vi "SID4.vi"() -> ()   [LabVIEW 2013]
uses:
  Program Files (x86)/SID4_SDK/SDKSID4_Types.llb/Refnum SDKSID4 session.ctl
  Shared/GUI_Template/GUI_master/tcp new data cluster.ctl
  <vilib>/vision/Image Controls.llb/IMAQ Image.ctl
  <vilib>/vision/NI_Vision_Development_Module.lvlib
  Shared/GUI_Template/GUI_master/tcp_new_data_event.ctl
  Program Files (x86)/SID4_SDK/SDKSID4_Types.llb/SDKSID4_Analysis info.ctl
  Program Files (x86)/SID4_SDK/SDKSID4_Types.llb/SDKSID4_Camera info.ctl
  Program Files (x86)/SID4_SDK/SDKSID4_Types.llb/SDKSID4_ImageCameraSize.ctl
panel:
  out "ROI Descriptor out":T1={"Global Rectangle"=[10, 10, 200, 200], "Contours"=[{"ID"=enum."External", "Type"=4, "Coordinates"=[10, 10, 200, 200]}]} {"Contours"."Type" items=["No Selection", "Point", "Line", "Rectangle", "Oval", "Polygon", "Free", "Annulus", "Unused2", "Unused3", "Broken Line", "Free Hand Line", "Rotated Rectangle"]}
  in  "pattern":string="*.png"
  in  "analyze folder":bool caption="sdfd"
  out "filenames":string[](array[string])
  in  "Folder to analyze":path=path "C:/Program Files (x86)/SID4_SDK/Examples/Mask files/Mask1.msk"
  in  "file?":bool caption="file (T) Live (F)"
  in  "save raw":bool caption="saves the intensity image retrieved from GEECS"
  in  "save measurement":bool caption="saves the recovered intensity and phase"
  in  "analyze":bool caption="analyzes the phase on either a file or the live image from GEECS"
  in  "continuous analysis":bool
  in  "Tab Control":T2(tab)
  in  "Profile path":path=path "C:/Users/loasis/Documents/000 Labview Local/Developers Version/Interface/GUI_SID4/profiles/SID4-034d default profile/SID4-034d default profile.txt"
  in  "Interferogram path":path=path "H:/data/p2/Y2014/09-Sep/14_0930/scans/Scan003/P2-phasics/Scan003_P2-phasics_047.png"
  in  "Reference Interferogram path":path=path "H:/data/p2/Y2014/09-Sep/14_0930/scans/Scan003/P2-phasics/Scan003_P2-phasics_001.png"
  in  "change reference":bool
  out "Saved Phase file":path
  out "Intensity file":path
  in  "GUIdevice 1":string="P2-phasics"
  in  "Tmp path":path=path "C:/Program Files (x86)/SID4_SDK/Examples/Interferograms/delete.tif"
  out "UnwrappingAlgoritm":u16(ring) items=["Basic", "Goldstein", "Lp-Norm"]
  out "UnwrappingOptions":u8[](array[numeric])
  out "Adv_Activation out":bool
  out "Adv_Niter":u16=10 caption="AdvAnalyse_# iterations out"
  out "Adv_MSE_Threshold":sgl=0.001 caption="AdvAnalyse_threshold out" format="%#.3e"
  in  "UnwrappingAlgoritm IN":u16(ring) items=["Basic", "Goldstein", "Lp-Norm"]
  in  "UnwrappingOptions IN":u8[](array[numeric])=[0, 0, 0, 0]
  in  "Adv_Activation in":bool
  in  "Adv_Niter 2":u16=10 caption="AdvAnalyse_# iterations in"
  in  "Adv_MSE_Threshold 2":sgl=0.001 caption="AdvAnalyse_threshold in" format="%#.3e"
  in  "change advanced parameters":bool caption="sdfd"
  out "image::1":T3(plugin-control) caption="Intensity"
  out "phasics-int1":T3(plugin-control)
  in  "change mask":bool
  in  "Tab Control 2":enum32{"Phase int graph", "Phase vision image"}(tab)
  out "PHASE":sgl[][](graph)
  out "phaseplot":T3(plugin-control)
  in  "Tab Control 3":enum32{"Intensity graph", "Phase lineout"}(tab)
  out "INTENSITY":sgl[][](graph)
  out "Line Profile":cluster{"x0":sgl, "dx":sgl, "Pixels Line":sgl[]}(graph)
  out "Line Information":T4 {"Standard Deviation" format="%#.2f"; "Mean" format="%#.2f"}
  out "SDKVersion":string
  out "Analysis info":T5
  out "Camera info":T6
  out "SNPhasics":string
  out "UserProfileDirectory":string
  out "UserProfile_LastReference":string
  out "UserProfileDescription":string
  out "UserProfile_File":string
  out "UserProfileName":string
  out "ImageCameraSize":T7
  in  "stop":bool
  out "tcp data event":T8
  out "error IO 2":errorcluster
  in  "MASK":T9(tab)
  in  "Mask path":path=path "C:/Program Files (x86)/SID4_SDK/Examples/Mask files/Mask1.msk"
  in  "ROI Descriptor IN":T1={"Global Rectangle"=[10, 10, 200, 200], "Contours"=[{"ID"=enum."External", "Type"=4, "Coordinates"=[10, 10, 200, 200]}]} {"Contours"."Type" items=["No Selection", "Point", "Line", "Rectangle", "Oval", "Polygon", "Free", "Annulus", "Unused2", "Unused3", "Broken Line", "Free Hand Line", "Rotated Rectangle"]}
  out "Current State":string
  # "Ensure paths in the profile path are correct to begin with or this program will not work!!!"
  # "Short term:\nfolder analysis\nrms deviation\n\n\nLong term:\nMode analysis\nAuto ROI based on intensity"
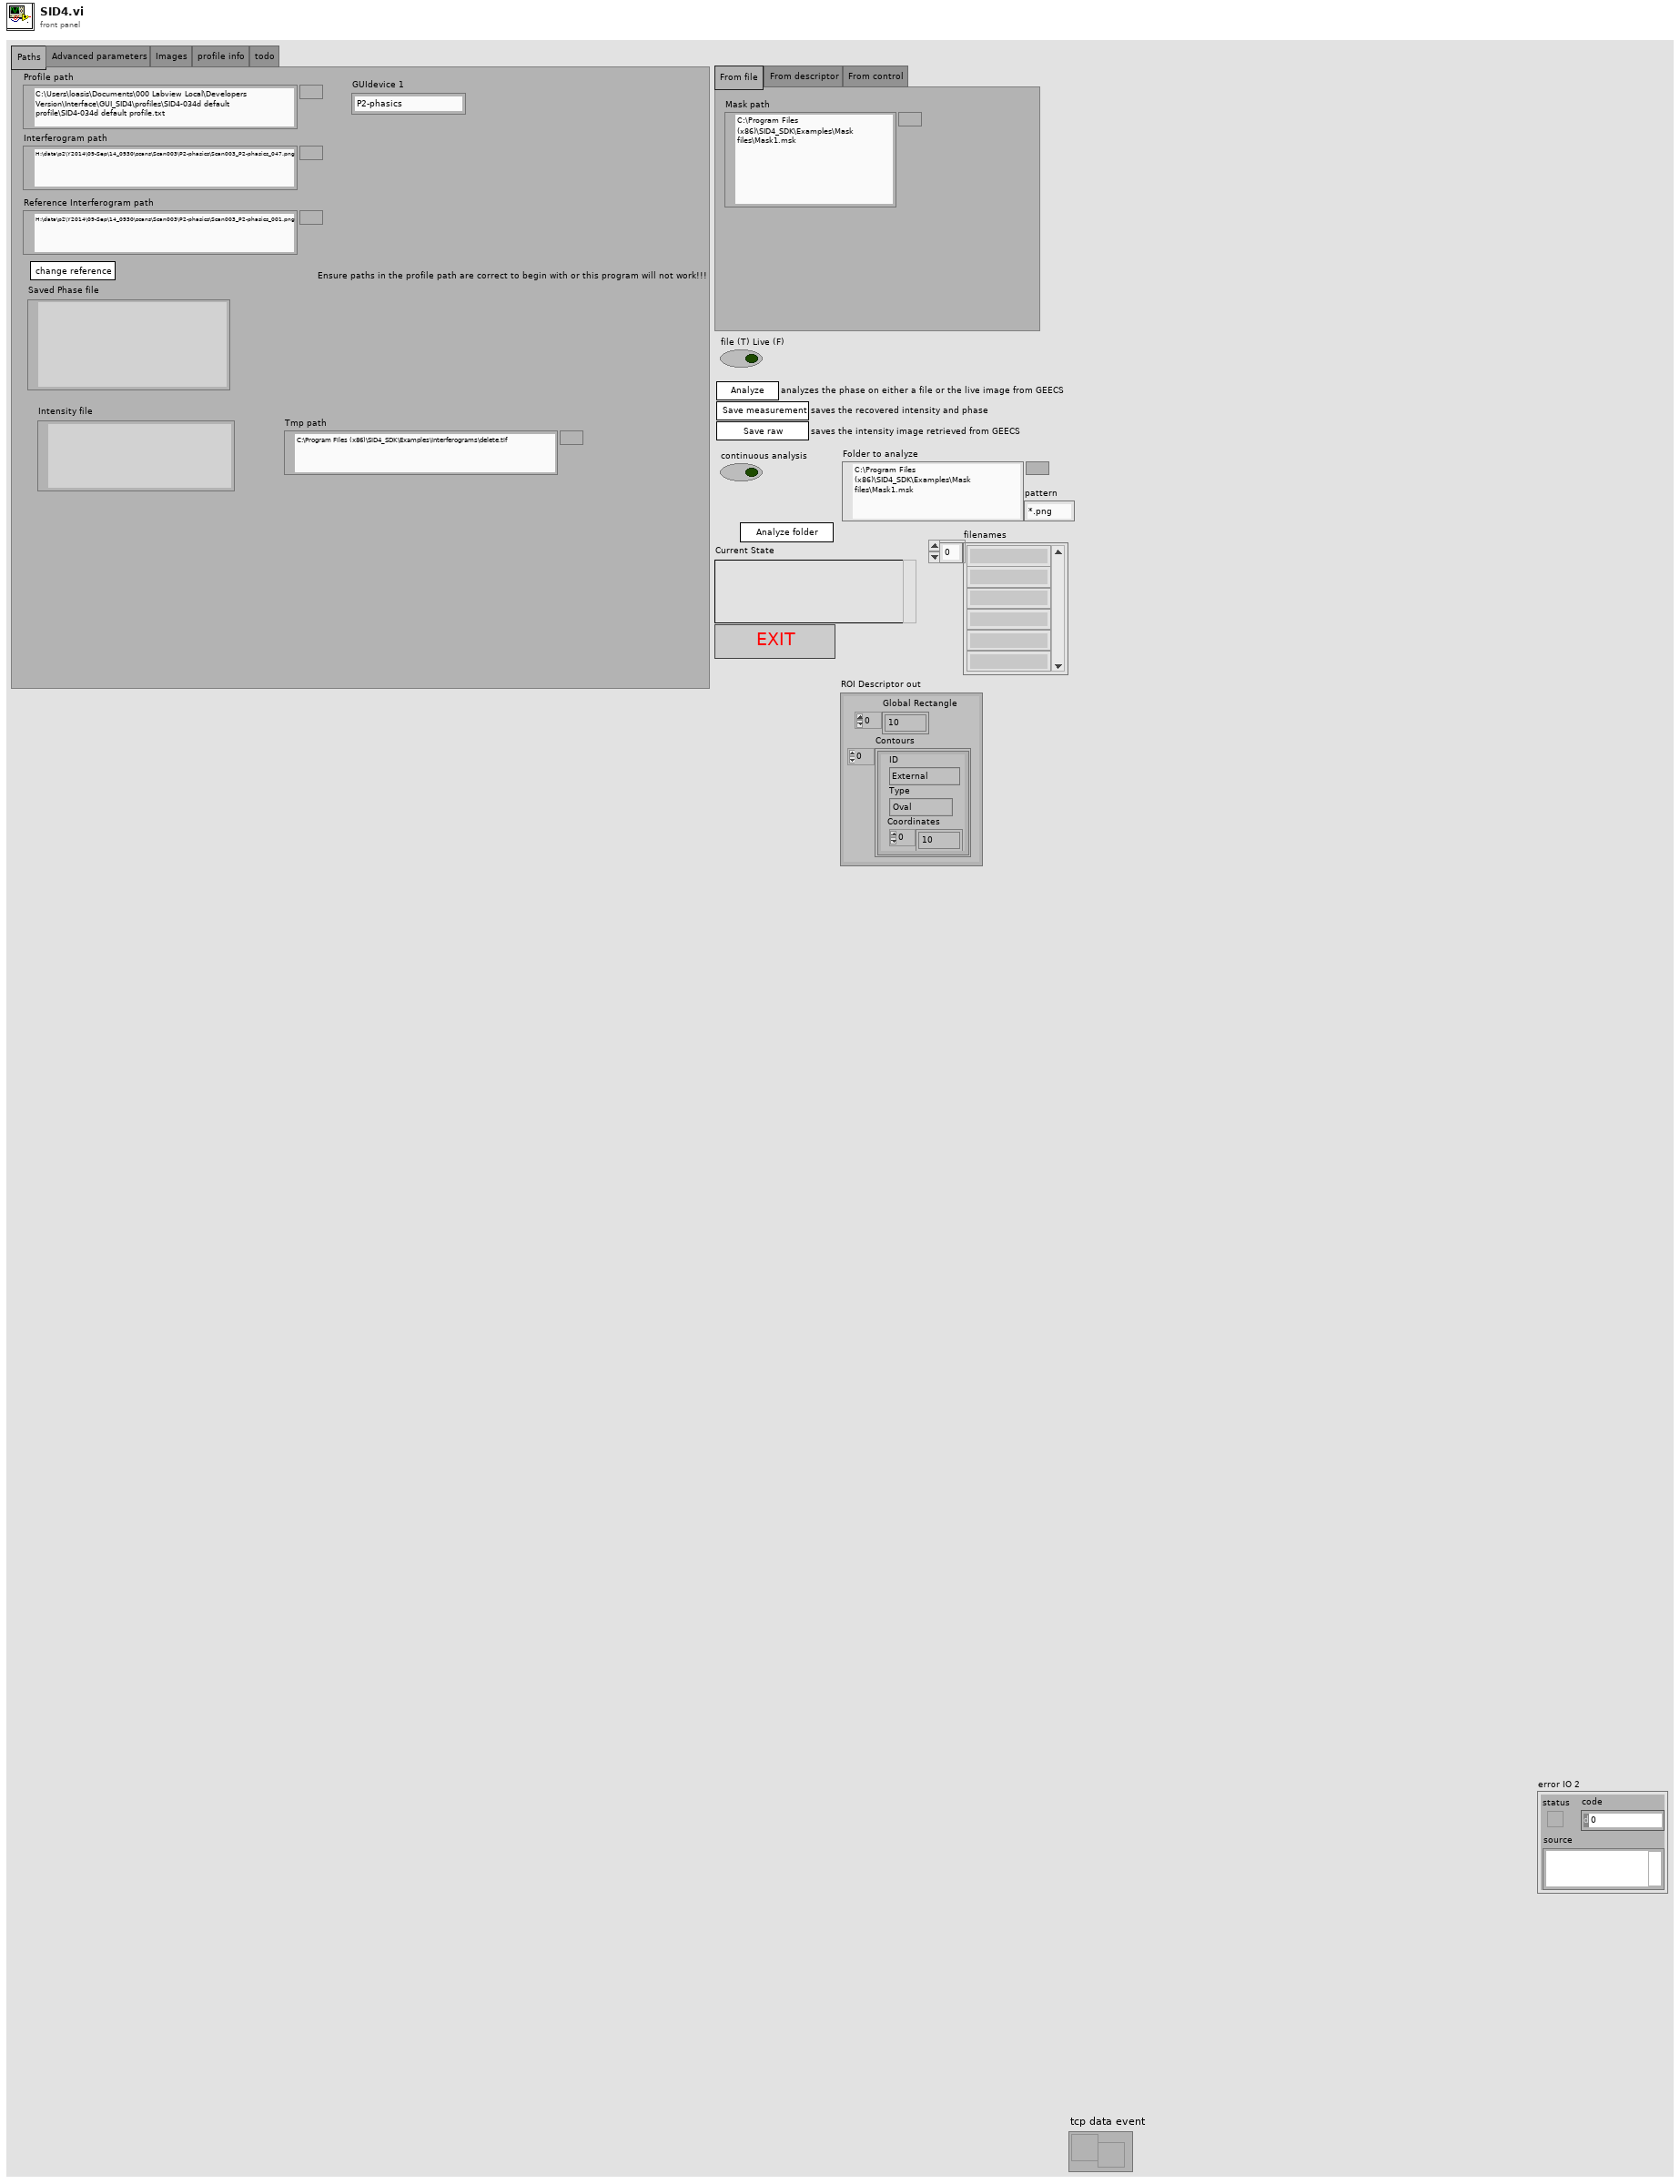
[diagram p1: front panel]
types:
  T1 = cluster{"Global Rectangle":i32[], "Contours":cluster{"ID":enum32{"External", "Internal"}, "Type":u32, "Coordinates":i32[]}[]}
  T2 = enum32{"Paths", "Advanced parameters", "Images", "profile info", "todo"}
  T3 = typedef "IMAQ Image.ctl" = refnum<image>
  T4 = cluster{"Minimum":sgl, "Maximum":sgl, "Mean":sgl, "Standard Deviation":sgl, "Count":i32}
  T5 = typedef "SDKSID4_Analysis info.ctl" = cluster{"Grating position (mm)":dbl, "wavelength (nm)":dbl, "Remove background image":bool, "PhaseSize_width":i32, "PhaseSize_Height":i32}
  T6 = typedef "SDKSID4_Camera info.ctl" = cluster{"Frame rate":i32, "Trigger mode":u32, "Gain":i32, "Exposure time":u32, "PixelSize(µm)":sgl, "NumberOfCameraRecorded":u8}
  T7 = typedef "SDKSID4_ImageCameraSize.ctl" = cluster{"nRow":i32, "nCol":i32}
  T8 = typedef "tcp_new_data_event.ctl" = refnum<user-event>
  T9 = enum32{"From file", "From descriptor", "From control"}
  T10 = typedef "tcp new data cluster.ctl" = cluster{"EventEnum":enum16{"new data", "connection status update"}, "Device name":string}
  T11 = enum32{"invalid app kind", "Development System", "Run Time System", "Student Edition", "Embedded LabVIEW", "Evaluation", "Custom"}
  T12 = typedef "Refnum SDKSID4 session.ctl" = refnum<k1>
  T13 = cluster{"Core":cluster{"Current VI Reference":refnum<vi>, "Close Panel on Exit?":bool}, "SDKSID4 sessionID":T12, "Interferogram path":path, "INTENSITY":sgl[][], "PHASE":sgl[][], "File paths":path[]}
  T14 = enum32{"Invalid", "Standard", "Closed", "Hidden", "Minimized", "Maximized"}
  T15 = typedef "Image Type" = u32
  T16 = cluster{"Global Rectangle":i32[], "Contours":cluster{"Contour Type":u32, "ROI Type":u32, "Points":i32[]}[]}
  T17 = cluster{"Min":sgl, "Max":sgl, "Mean":sgl, "Std Dev":sgl, "Count":i32}
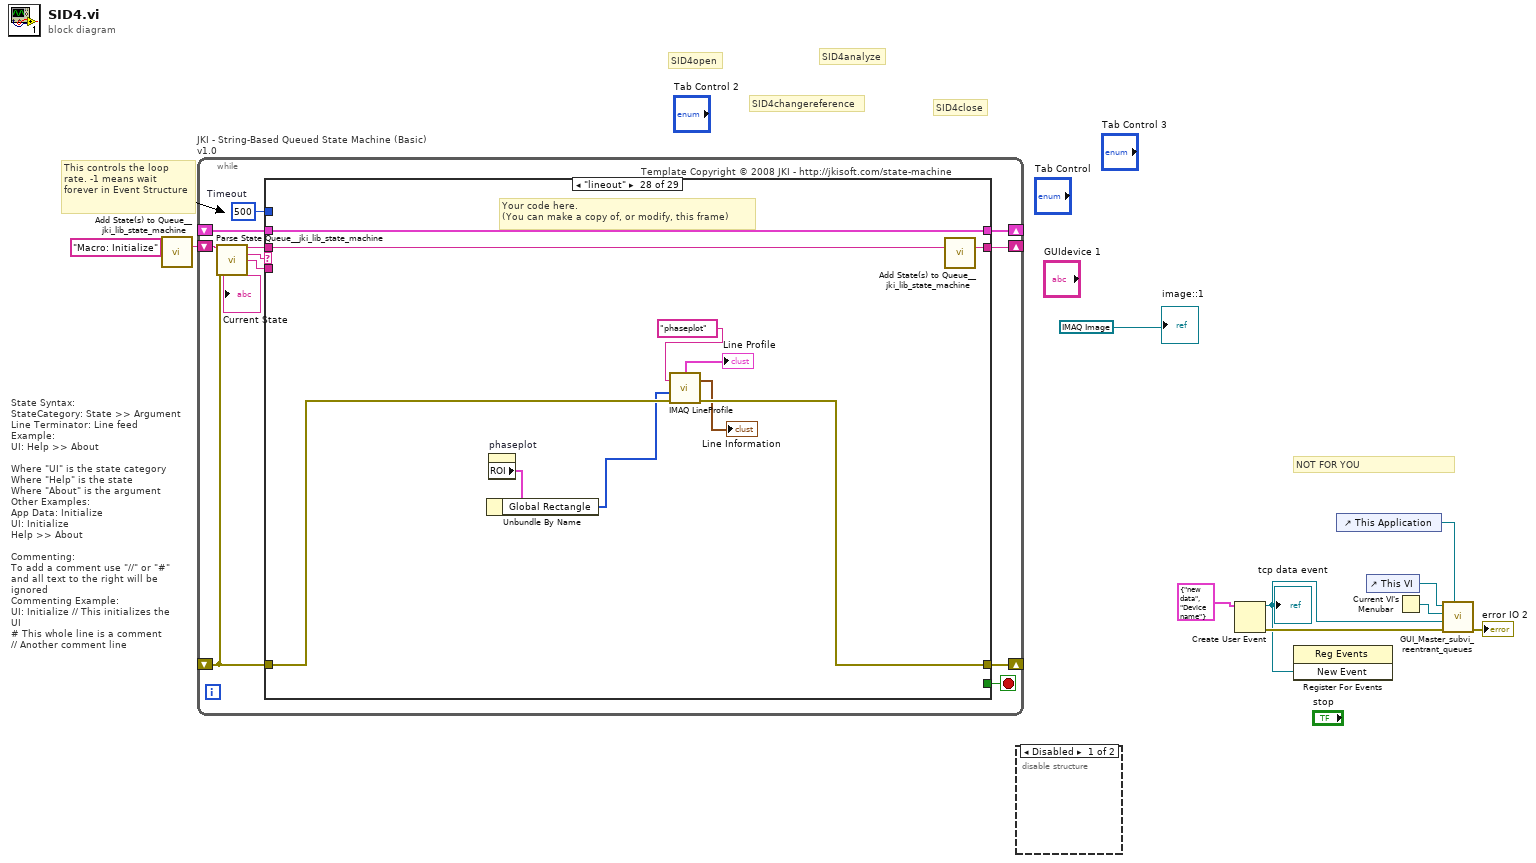
[diagram p0: block diagram]
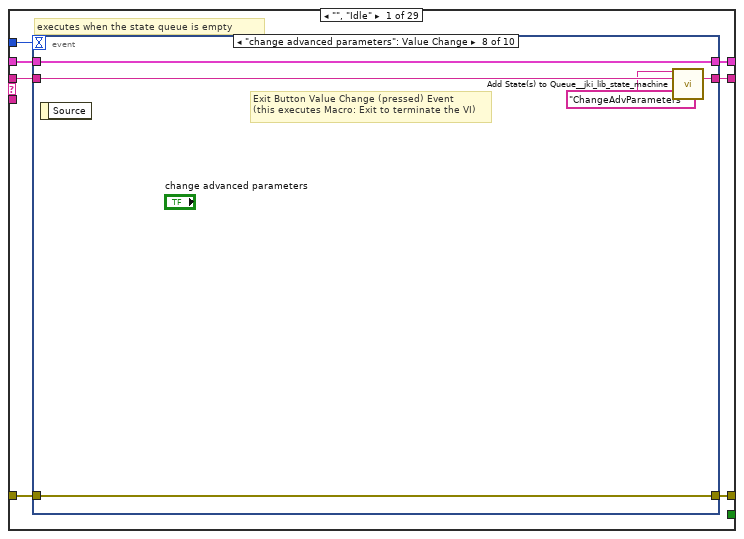
[diagram p3: hidden frame]
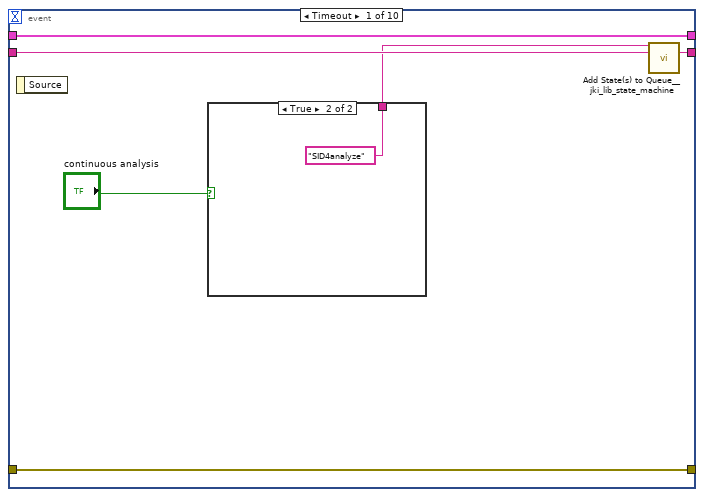
[diagram p4: hidden frame]
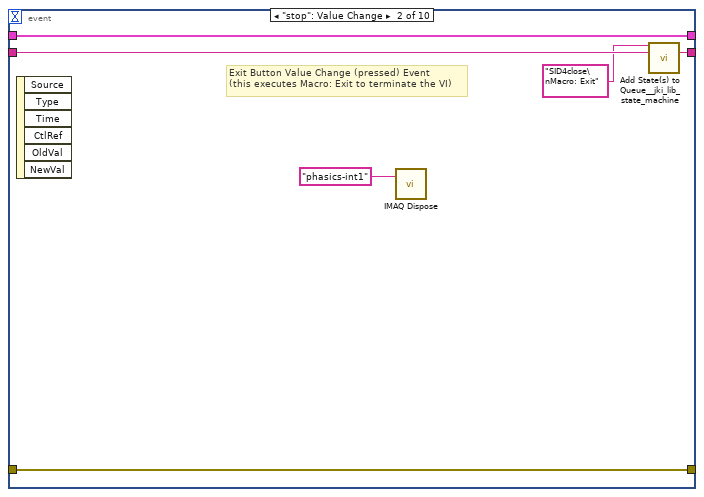
[diagram p6: hidden frame]
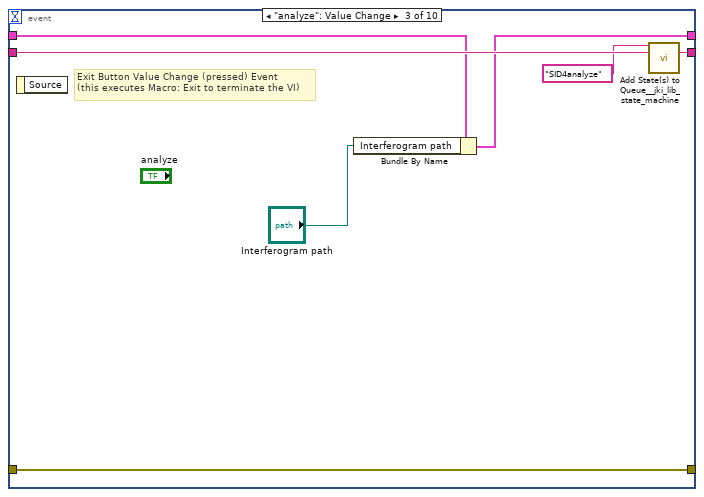
[diagram p7: hidden frame]
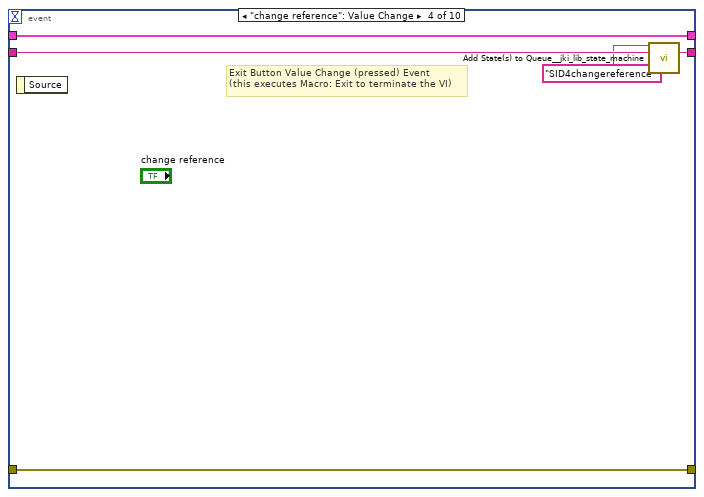
[diagram p8: hidden frame]
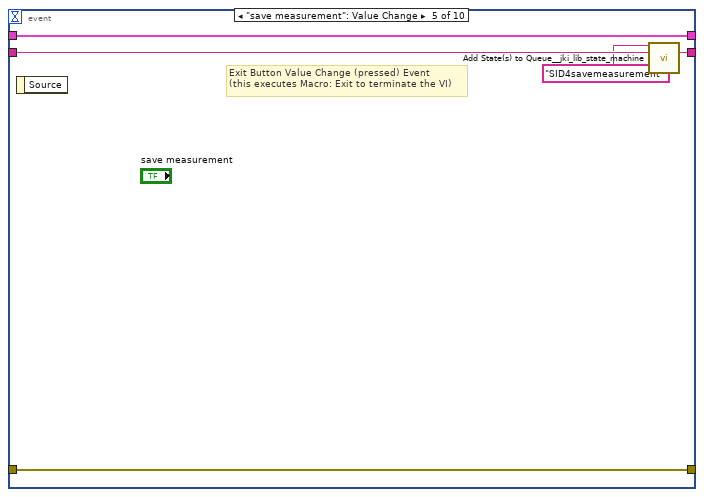
[diagram p9: hidden frame]
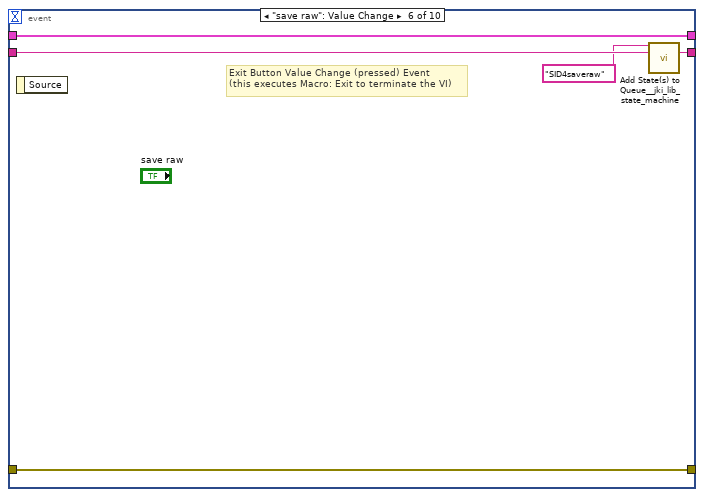
[diagram p10: hidden frame]
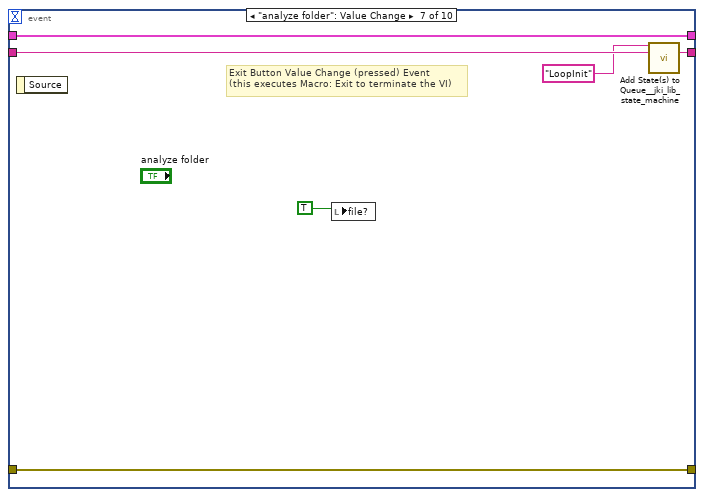
[diagram p11: hidden frame]
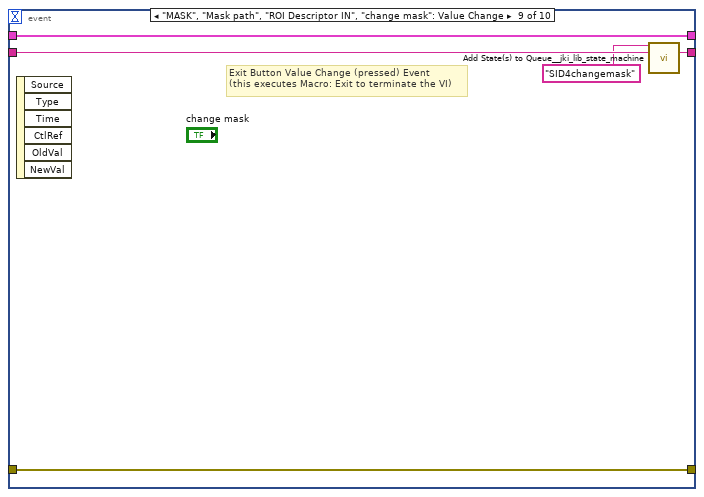
[diagram p12: hidden frame]
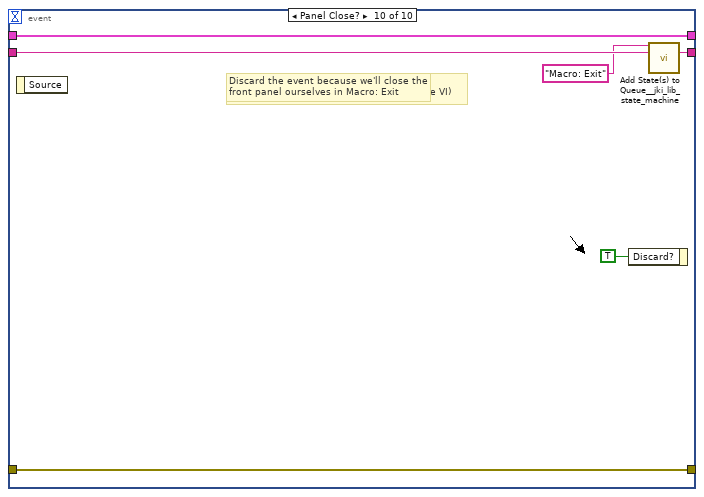
[diagram p13: hidden frame]
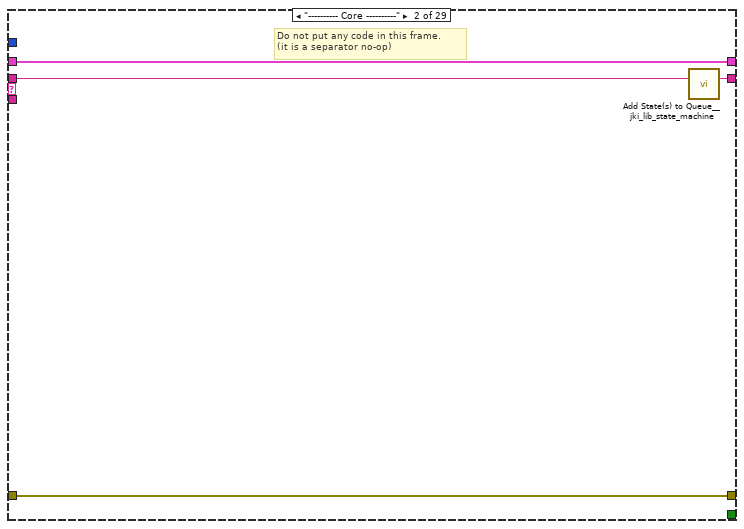
[diagram p14: hidden frame]
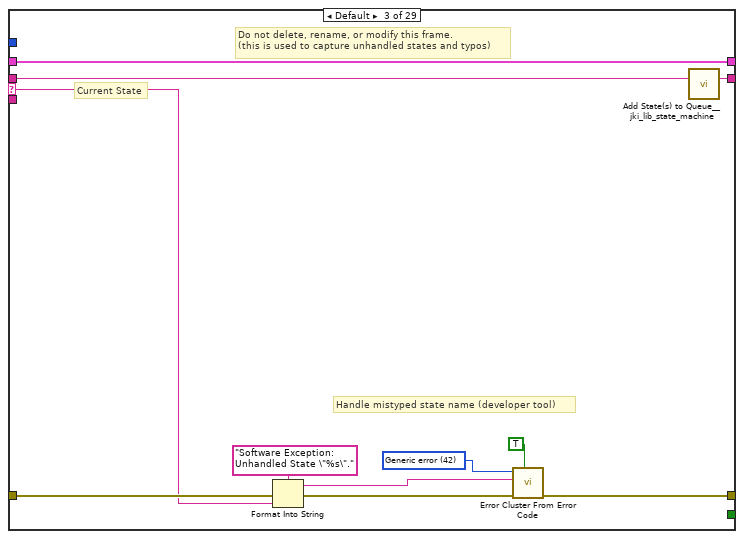
[diagram p15: hidden frame]
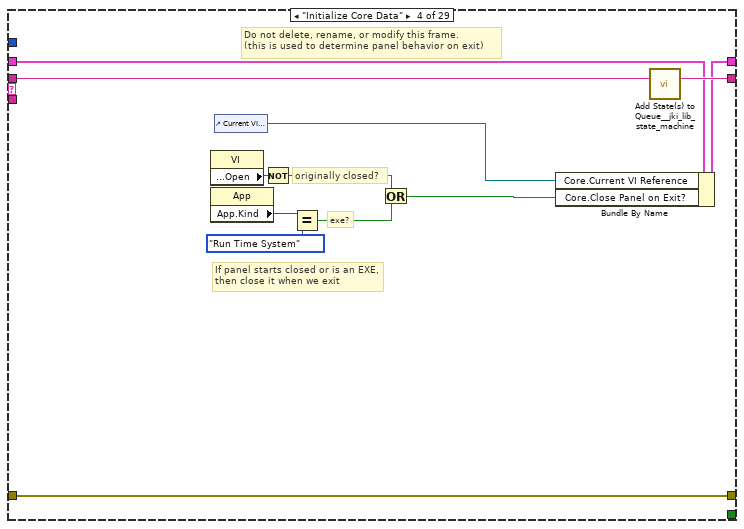
[diagram p16: hidden frame]
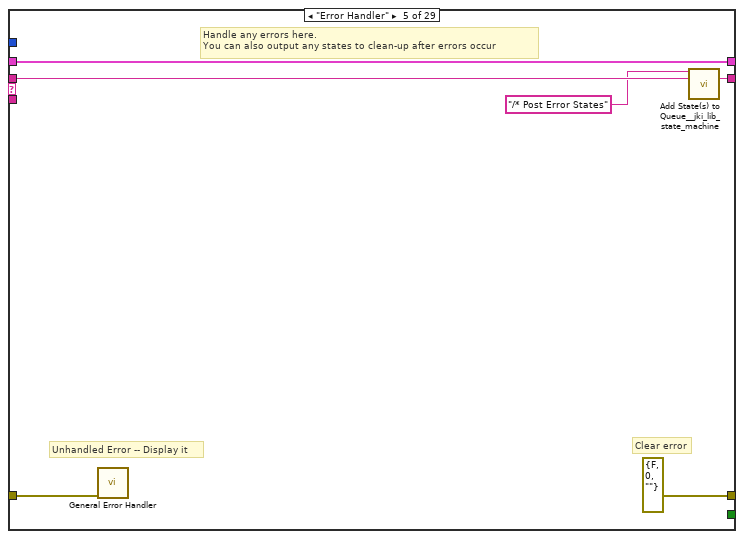
[diagram p17: hidden frame]
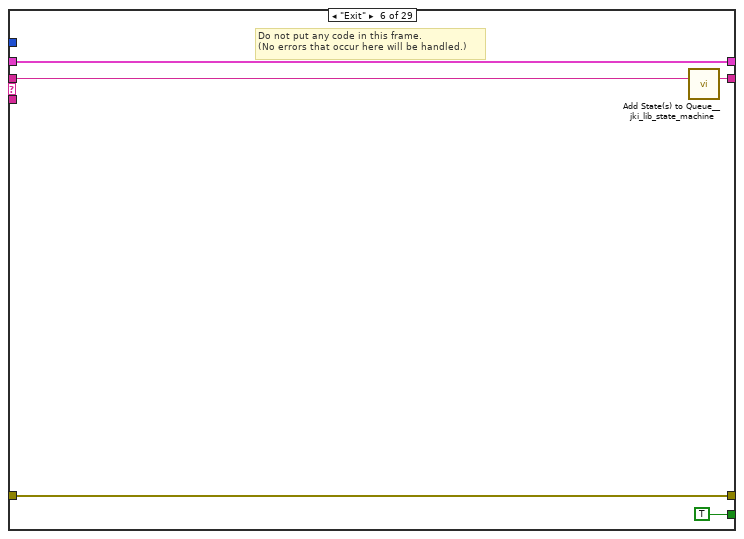
[diagram p18: hidden frame]
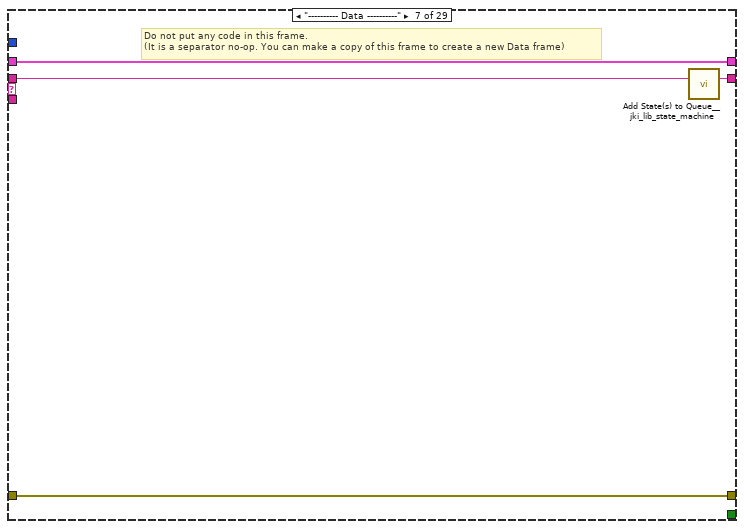
[diagram p19: hidden frame]
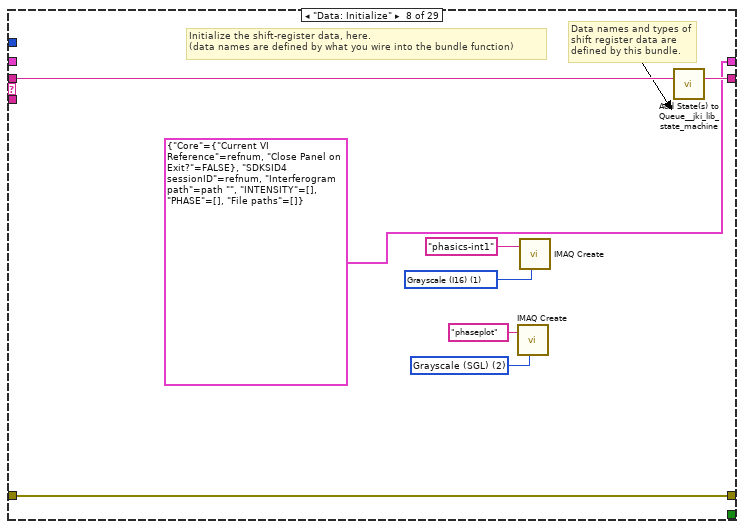
[diagram p20: hidden frame]
diagram:
  # "NOT FOR YOU"
  # "SID4close"
  # "SID4changereference"
  # "SID4analyze"
  # "SID4open"
  # "State Syntax:\nStateCategory: State >> Argument\nLine Terminator: Line feed\nExample:\nUI: Help >> About\n\nWhere \"UI\" is the state category\nWhere \"Help\" is the state\nWhere \"About\" is the argument\nOther Examples:\nApp Data: Initialize\nUI: Initialize\nHelp >> About\n\nCommenting:\nTo add a comment use \"//\" or \"#\" and all text to the right will be ignored\nCommenting Example:\nUI: Initialize // This initializes the UI\n# This whole line is a comment\n// Another comment line"
  # "This controls the loop rate. -1 means wait forever in Event Structure"
  n1 = call <vilib>:"Add State(s) to Queue__jki_lib_state_machine.vi"("State(s) in (\"\")"="Macro: Initialize") -> ("States Out"=w10:string)  [unwired: 14 in]
  n2 = while "JKI - String-Based Queued State Machine (Basic) v1.0" {
    shift-right: [w14] -> _
    shift-left: _ -> [w13]
    shift-right: [w17] -> _
    shift-left: _ -> [w11]
    shift-right: [w16] -> _
    shift-left: w10 -> [w18]
    stop <- w15 stop-if-true
    w12 = 500  # Timeout
    # "Template Copyright © 2008 JKI - http://jkisoft.com/state-machine"
    n3 = call <vilib>:"Parse State Queue__jki_lib_state_machine.vi"("State Queue"=w18, "Error In (no error)"=w11) -> ("Remaining States"=w20:string, "Current State"=w21:string, "Arguments"=w19:string)  [unwired: 11 in]
    "Current State" <- w21
    n4 = case shown="\"lineout\"" w21 {
      selector: w21 -> [_ _ w90 _ _ _ _ _ _ _ _ _ _ _ _ _ _ _ _ _ _ _ _ _ _ _ _ _ _]
      tunnel: w20 -> [w28 w89 w94 w112 w118 w123 w127 w135 w141 w145 w149 w155 w166 w192 w197 w207 w211 w218 w249 w300 w305 w317 w351 w358 w374 w386 w415 w425 w429]
      tunnel: w19 -> [_ _ _ _ _ _ _ _ _ _ _ w150 w160 _ _ _ _ _ _ _ _ _ _ _ _ _ _ _ _]
      tunnel: w13 -> [w26 w86 w92 w103 w115 w121 w124 _ w136 w142 w147 w153 w162 w189 w194 w204 w208 w215 w245 w294 w303 w315 w349 w356 w366 w380 w399 w423 w426]
      tunnel: [w25 w87 w96 w109 errorcluster {"status"=FALSE, "code"=0, "source"=""} ("error out") w120 w125 w133 w137 w143 w146 w151 w163 w190 w195 w205 w209 w213 w240 w295 w301 w311 w346 w353 w372 w384 w396 w421 w427] -> w17
      tunnel: w11 -> [w24 w87 w95 w109 w114 w120 w125 w133 w138 w143 w146 w152 w164 w190 w195 w205 w209 w216 w246 w296 w302 w312 w345 w354 w372 w384 w397 w422 w427]
      tunnel: [w27 w88 w93 w111 w117 w122 w126 w134 w140 w144 w148 w154 w165 w191 w196 w206 w210 w217 w248 w299 w304 w316 w350 w357 w373 w385 w414 w424 w428] -> w16
      tunnel: [_ _ _ _ _ TRUE _ _ _ _ _ _ _ _ _ _ _ _ _ _ _ _ _ _ _ _ _ _ _] -> w15
      tunnel: [w23 w86 w92 w110 w115 w121 w124 T13 {"Core"={"Current VI Reference"=refnum, "Close Panel on Exit?"=FALSE}, "SDKSID4 sessionID"=refnum, "Interferogram path"=path "", "INTENSITY"=[], "PHASE"=[], "File paths"=[]} w136 w142 w147 w153 w162 w189 w194 w204 w208 w214 w244 w294 w303 w315 w349 w356 w365 w379 w399 w423 w426] -> w14
      tunnel: w12 -> [w22 _ _ _ _ _ _ _ _ _ _ _ _ _ _ _ _ _ _ _ _ _ _ _ _ _ _ _ _]
      frame "", "Idle" {
        # "executes when the state queue is empty"
        n5 = event shown="[7] \"change advanced parameters\": Value Change" {
          selector: _ -> [_ _ _ _ _ _ _ _ _ _]
          dyn-events: _ -> [_ _ _ _ _ _ _ _ _ _]
          timeout: w22 -> [_ _ _ _ _ _ _ _ _ _]
          tunnel: w28 -> [w34 w41 w48 w53 w58 w63 w69 w74 w79 w85]
          tunnel: [w33 w40 w47 w52 w57 w62 w68 w73 w78 w84] -> w27
          tunnel: w26 -> [w31 w38 w44 w50 w55 w60 w66 w71 w76 w82]
          tunnel: [w32 w39 w46 w51 w56 w61 w67 w72 w77 w83] -> w25
          tunnel: w24 -> [w32 w39 w46 w51 w56 w61 w67 w72 w77 w83]
          tunnel: [w31 w38 w43 w50 w55 w60 w66 w71 w76 w82] -> w23
          event Timeout {
            n6 = event-data() -> ()  [unwired: 1 in, 1 out]
            n7 = case shown="True" "continuous analysis" {
              tunnel: [_ "SID4analyze" ("State(s) in Front (\"\")")] -> w29
              frame False {
              }
              frame True {
              }
            }
            n8 = call <vilib>:"Add State(s) to Queue__jki_lib_state_machine.vi"("State(s) in Front (\"\")"=w29, "State(s) in (\"\")"=w34) -> ("States Out"=w33:string)  [unwired: 13 in]
          }
          event "stop": Value Change {
            # "Exit Button Value Change (pressed) Event\n(this executes Macro: Exit to terminate the VI)"
            n9 = event-data() -> ()  [unwired: 1 in, 6 out]
            n10 = call "IMAQ Dispose"("Image"="phasics-int1" ("Image Name")) -> ()  [unwired: 5 in, 1 out]
            n11 = call <vilib>:"Add State(s) to Queue__jki_lib_state_machine.vi"("State(s) in Front (\"\")"="SID4close\nMacro: Exit", "State(s) in (\"\")"=w41) -> ("States Out"=w40:string)  [unwired: 13 in]
          }
          event "analyze": Value Change {
            # "Exit Button Value Change (pressed) Event\n(this executes Macro: Exit to terminate the VI)"
            n12 = event-data() -> ()  [unwired: 1 in, 1 out]
            n13 = Bundle By Name(cluster=w44, "Interferogram path"="Interferogram path") -> (w43:T13)
            n14 = call <vilib>:"Add State(s) to Queue__jki_lib_state_machine.vi"("State(s) in Front (\"\")"="SID4analyze", "State(s) in (\"\")"=w48) -> ("States Out"=w47:string)  [unwired: 13 in]
          }
          event "change reference": Value Change {
            # "Exit Button Value Change (pressed) Event\n(this executes Macro: Exit to terminate the VI)"
            n15 = event-data() -> ()  [unwired: 1 in, 1 out]
            n16 = call <vilib>:"Add State(s) to Queue__jki_lib_state_machine.vi"("State(s) in Front (\"\")"="SID4changereference", "State(s) in (\"\")"=w53) -> ("States Out"=w52:string)  [unwired: 13 in]
          }
          event "save measurement": Value Change {
            # "Exit Button Value Change (pressed) Event\n(this executes Macro: Exit to terminate the VI)"
            n17 = event-data() -> ()  [unwired: 1 in, 1 out]
            n18 = call <vilib>:"Add State(s) to Queue__jki_lib_state_machine.vi"("State(s) in Front (\"\")"="SID4savemeasurement", "State(s) in (\"\")"=w58) -> ("States Out"=w57:string)  [unwired: 13 in]
          }
          event "save raw": Value Change {
            # "Exit Button Value Change (pressed) Event\n(this executes Macro: Exit to terminate the VI)"
            n19 = event-data() -> ()  [unwired: 1 in, 1 out]
            n20 = call <vilib>:"Add State(s) to Queue__jki_lib_state_machine.vi"("State(s) in Front (\"\")"="SID4saveraw", "State(s) in (\"\")"=w63) -> ("States Out"=w62:string)  [unwired: 13 in]
          }
          event "analyze folder": Value Change {
            # "Exit Button Value Change (pressed) Event\n(this executes Macro: Exit to terminate the VI)"
            n21 = event-data() -> ()  [unwired: 1 in, 1 out]
            n22 = local write "file?"(TRUE ("file?")) -> ()
            n23 = call <vilib>:"Add State(s) to Queue__jki_lib_state_machine.vi"("State(s) in Front (\"\")"="LoopInit", "State(s) in (\"\")"=w69) -> ("States Out"=w68:string)  [unwired: 13 in]
          }
          event "change advanced parameters": Value Change {
            # "Exit Button Value Change (pressed) Event\n(this executes Macro: Exit to terminate the VI)"
            n24 = event-data() -> ()  [unwired: 1 in, 1 out]
            n25 = call <vilib>:"Add State(s) to Queue__jki_lib_state_machine.vi"("State(s) in Front (\"\")"="ChangeAdvParameters", "State(s) in (\"\")"=w74) -> ("States Out"=w73:string)  [unwired: 13 in]
          }
          event "MASK", "Mask path", "ROI Descriptor IN", "change mask": Value Change {
            # "Exit Button Value Change (pressed) Event\n(this executes Macro: Exit to terminate the VI)"
            n26 = event-data() -> ()  [unwired: 1 in, 6 out]
            n27 = call <vilib>:"Add State(s) to Queue__jki_lib_state_machine.vi"("State(s) in Front (\"\")"="SID4changemask", "State(s) in (\"\")"=w79) -> ("States Out"=w78:string)  [unwired: 13 in]
          }
          event Panel Close? {
            # "Discard the event because we'll close the front panel ourselves in Macro: Exit"
            # "Close Panel button (pressed) Event\n(this executes Macro: Exit to terminate the VI)"
            n28 = event-data() -> ()  [unwired: 1 in, 1 out]
            n29 = event-data("Discard?"=TRUE) -> ()  [unwired: 1 in, 1 out]
            n30 = call <vilib>:"Add State(s) to Queue__jki_lib_state_machine.vi"("State(s) in Front (\"\")"="Macro: Exit", "State(s) in (\"\")"=w85) -> ("States Out"=w84:string)  [unwired: 13 in]
          }
        }
      }
      frame "---------- Core ----------" {
        # "Do not put any code in this frame.\n(it is a separator no-op)"
        n31 = call <vilib>:"Add State(s) to Queue__jki_lib_state_machine.vi"("State(s) in (\"\")"=w89) -> ("States Out"=w88:string)  [unwired: 14 in]
      }
      frame Default {
        w99 = 42 items=["No error", "Argument error", "Memory is full", "Out of zone", "End of file", "File already open", "Generic file I/O error", "File not found", "File permission error", "Disk is full", "Duplicate path", "Too many files open", "System feature not enabled", "Resource file not found", "Cannot add resource", "Resource not found", "Image not found", "Image memory error", "Pen does not exist", "Config type invalid", "Config token not found", "Config parse error", "Config memory error", "Bad external code format", "Bad external code offset", "External code not present", "Null window", "Destroy window error", "Null menu", "Print aborted", "Bad print record", "Print driver error", "Windows error during printing", "Memory error during printing", "Print dialog error", "Generic print error", "Invalid device refnum", "Device not found", "Device parameter error", "Device unit error", "Cannot open device", "Device call aborted", "Generic error", "Cancelled by user", "Object ID too low", "Object ID too high", "Object not in heap", "Unknown heap", "Unknown object (invalid DefProc)", "Unknown object (DefProc not in table)", "Message out of range", "Invalid (null) method", "Unknown message", "Manager call not supported", "Bad address", "Network operation in progress", "Network operation timed out", "Connection is busy", "Network attribute not supported", "Network error", "Address in use", "System out of memory", "Connection aborted", "Connection refused", "Not connected", "Already connected", "Connection closed", "Initialization error (interapplication manager)", "Bad occurrence", "Wait on unbound occurrence handler", "Occurrence queue overflow", "Datalog type conflict", "Unused", "Unrecognized type (interapplication manager)", "Memory corrupt", "Failed to make temporary DLL", "Old CIN version", "Drag socket not found", "Failed to load drop-object", "Failed to register OLE object", "Failed to release OLE object", "Format specifier type mismatch", "Unknown format specifier", "Too few format specifiers", "Too many format specifiers", "Scan failed", "Newer CIN version", "Error converting to variant", "Runtime menu error", "Password tampered", "Variant attribute not found", "Incompatible variant data type", "Event data is not available", "Event Store is not present", "Occurrence is not found", "Event Queue is not created", "Event info is not available", "Refnum passed is NULL", "Error retrieving Class GUID", "Error retrieving CoClass GUID", "Error retrieving TypeLib GUID.", "Bad built application magic bytes.", "Specific driver is different from the specific driver associated with the Logical Name.", "There is no session opened to the class driver.", "Max Error", "MAX - Error with config objects", "MAX - Error loading configuration", "MAX - Group not supported"]
        # "Current State"
        # "Do not delete, rename, or modify this frame.\n(this is used to capture unhandled states and typos)"
        # "Handle mistyped state name (developer tool)"
        n32 = Format Into String(format string="Software Exception: Unhandled State \"%s\"." ("message"), error in=w95, w90) -> (resulting string=w98:string, error out=w97:errorcluster)  [unwired: 1 in]
        n33 = call <vilib>:"Error Cluster From Error Code.vi"("show call chain? (False)"=TRUE, "error in (no error)"=w97, "error message (\"\")"=w98, "error code (0)"=w99) -> ("error out"=w96:errorcluster)  [unwired: 5 in]
        n34 = call <vilib>:"Add State(s) to Queue__jki_lib_state_machine.vi"("State(s) in (\"\")"=w94) -> ("States Out"=w93:string)  [unwired: 14 in]
      }
      frame "Initialize Core Data" {
        # "Do not delete, rename, or modify this frame.\n(this is used to determine panel behavior on exit)"
        # "originally closed?"
        # "exe?"
        # "If panel starts closed or is an EXE, then close it when we exit"
        n35 = property class="VI"() -> ("Front Panel.Open"=w108:bool)  [unwired: 2 in, 2 out]
        n36 = property class="App"() -> ("App.Kind"=w107:T11)  [unwired: 2 in, 2 out]
        n37 = control-ref of="Current VI Reference"() -> (w101:refnum<vi>)
        n38 = Not(x=w108) -> (.not. x?=w105:bool)
        n39 = Equal?(x=w107, y=T11."Run Time System" ("Application:Kind")) -> (x = y?=w104:bool)
        n40 = Or(x=w105, y=w104) -> (x .or. y?=w102:bool)
        n41 = Bundle By Name(cluster=w103, "Core.Current VI Reference"=w101, "Core.Close Panel on Exit?"=w102) -> (w110:T13)
        n42 = call <vilib>:"Add State(s) to Queue__jki_lib_state_machine.vi"("State(s) in (\"\")"=w112) -> ("States Out"=w111:string)  [unwired: 14 in]
      }
      frame "Error Handler" {
        # "Unhandled Error -- Display it"
        # "Handle any errors here.\nYou can also output any states to clean-up after errors occur"
        # "Clear error"
        n43 = call <vilib>:"General Error Handler.vi"("error in (no error)"=w114) -> ()  [unwired: 10 in, 5 out]
        n44 = call <vilib>:"Add State(s) to Queue__jki_lib_state_machine.vi"("State(s) in Front (\"\")"="/* Post Error States", "State(s) in (\"\")"=w118) -> ("States Out"=w117:string)  [unwired: 13 in]
      }
      frame "Exit" {
        # "Do not put any code in this frame.\n(No errors that occur here will be handled.)"
        n45 = call <vilib>:"Add State(s) to Queue__jki_lib_state_machine.vi"("State(s) in (\"\")"=w123) -> ("States Out"=w122:string)  [unwired: 14 in]
      }
      frame "---------- Data ----------" {
        # "Do not put any code in this frame.\n(It is a separator no-op. You can make a copy of this frame to create a new Data frame)"
        n46 = call <vilib>:"Add State(s) to Queue__jki_lib_state_machine.vi"("State(s) in (\"\")"=w127) -> ("States Out"=w126:string)  [unwired: 14 in]
      }
      frame "Data: Initialize" {
        w128 = T15 2 items=["Grayscale (U8)", "Grayscale (I16)", "Grayscale (SGL)", "Complex (CSG)", "RGB (U32)", "HSL (U32)", "RGB (U64)", "Grayscale (U16)"] ("Image Type")
        w130 = T15 1 items=["Grayscale (U8)", "Grayscale (I16)", "Grayscale (SGL)", "Complex (CSG)", "RGB (U32)", "HSL (U32)", "RGB (U64)", "Grayscale (U16)"] ("Image Type")
        # "Data names and types of shift register data are defined by this bundle."
        # "Initialize the shift-register data, here.\n(data names are defined by what you wire into the bundle function)"
        n47 = call "IMAQ Create"("Image Name"="phaseplot", "Image Type"=w128) -> ()  [unwired: 3 in, 2 out]
        n48 = call "IMAQ Create"("Image Name"="phasics-int1", "Image Type"=w130) -> ()  [unwired: 3 in, 2 out]
        n49 = call <vilib>:"Add State(s) to Queue__jki_lib_state_machine.vi"("State(s) in (\"\")"=w135) -> ("States Out"=w134:string)  [unwired: 14 in]
      }
      frame "Data: Cleanup" {
        # "Cleanup any data and references, here.\n(this is called automatically, by the Macro: Exit)"
        n50 = Unbundle By Name(w136) -> ("Core.Current VI Reference"=w139:refnum<vi>)
        n51 = Close Reference(reference=w139, error in (no error)=w138) -> (error out=w137:errorcluster)
        n52 = call <vilib>:"Add State(s) to Queue__jki_lib_state_machine.vi"("State(s) in (\"\")"=w141) -> ("States Out"=w140:string)  [unwired: 14 in]
      }
      frame "---------- UI ----------" {
        # "Do not put any code in this frame.\n(It is a separator no-op. You can make a copy of this frame to create a new UI frame)"
        n53 = call <vilib>:"Add State(s) to Queue__jki_lib_state_machine.vi"("State(s) in (\"\")"=w145) -> ("States Out"=w144:string)  [unwired: 14 in]
      }
      frame "UI: Initialize" {
        # "Initialize the User Interface, here.\n(this is called automatically, by the Macro: Init)"
        n54 = call <vilib>:"Add State(s) to Queue__jki_lib_state_machine.vi"("State(s) in (\"\")"=w149) -> ("States Out"=w148:string)  [unwired: 14 in]
      }
      frame "UI: Cursor Set" {
        # "Argument"
        # "Set and Unset Cursor Busy.\n(Usage: \"UI: Cursor Set >> Busy|Idle\")"
        n55 = case shown="\"Idle\", Default" w150 {
          tunnel: w152 -> [w157 w159]
          tunnel: [w156 w158] -> w151
          frame "Idle", Default {
            n56 = call <vilib>:"Unset Busy.vi"("error in (no error)"=w157) -> ("error out"=w156:errorcluster)  [unwired: 10 in]
          }
          frame "Busy" {
            n57 = call <vilib>:"Set Busy.vi"("error in (no error)"=w159) -> ("error out"=w158:errorcluster)  [unwired: 9 in, 1 out]
          }
        }
        n58 = call <vilib>:"Add State(s) to Queue__jki_lib_state_machine.vi"("State(s) in (\"\")"=w155) -> ("States Out"=w154:string)  [unwired: 14 in]
      }
      frame "UI: Front Panel State" {
        # "Argument"
        # "Set Front Panel Open or Closed\n(Usage: \"UI: Front Panel State >> Open|Close\")"
        n59 = Unbundle By Name(w162) -> ("Core.Current VI Reference"=w161:refnum<vi>)
        n60 = case shown="\"Open\", Default" w160 {
          tunnel: w164 -> [w170 w183]
          tunnel: [w172 w184] -> w163
          tunnel: w161 -> [w171 w181]
          frame "Open", Default {
            n61 = property class="VI"(reference=w171, error in=w170) -> (reference out=w168:refnum<vi>, error out=w169:errorcluster, "Front Panel.Open"=w167:bool)
            n62 = case shown="False" w167 {
              tunnel: [w175 w178] -> w172
              tunnel: w169 -> [w174 w178]
              tunnel: w168 -> [w173 _]
              frame False {
                n63 = invoke class="VI" method="FP.Open"(reference=w173, error in=w174, "Activate"=TRUE, "State"=T14."Standard") -> (error out=w175:errorcluster)  [unwired: 1 in, 4 out]
              }
              frame True {
              }
            }
          }
          frame "Close" {
            n64 = property class="VI"(reference=w181, error in=w183) -> (reference out=w180:refnum<vi>, error out=w182:errorcluster, "Front Panel.Open"=w179:bool)
            n65 = case shown="True" w179 {
              tunnel: [w185 w188] -> w184
              tunnel: w182 -> [w185 w187]
              tunnel: w180 -> [_ w186]
              frame False {
              }
              frame True {
                n66 = invoke class="VI" method="FP.Close"(reference=w186, error in=w187) -> (error out=w188:errorcluster)  [unwired: 1 in, 2 out]
              }
            }
          }
        }
        n67 = call <vilib>:"Add State(s) to Queue__jki_lib_state_machine.vi"("State(s) in (\"\")"=w166) -> ("States Out"=w165:string)  [unwired: 14 in]
      }
      frame "---------- Macro ----------" {
        # "Do not put any code in this frame.\n(It is a separator no-op. You can make a copy of this frame to create a new Macro frame)"
        n68 = call <vilib>:"Add State(s) to Queue__jki_lib_state_machine.vi"("State(s) in (\"\")"=w192) -> ("States Out"=w191:string)  [unwired: 14 in]
      }
      frame "Macro: Initialize" {
        w193 = "Data: Initialize\nInitialize Core Data\nUI: Initialize\nUI: Front Panel State >> Open\nSID4open"  # Data: Initialize Initialize Core Data UI: Initialize UI: Front Panel State >> Open SID4open
        # "Initialization Macro\n(This is called once, when the VI starts)"
        n69 = call <vilib>:"Add State(s) to Queue__jki_lib_state_machine.vi"("State(s) in Front (\"\")"=w193, "State(s) in (\"\")"=w197) -> ("States Out"=w196:string)  [unwired: 13 in]
      }
      frame "Macro: Exit" {
        # "Exit Macro\n(This is called once, when the VI exits)"
        n70 = Unbundle By Name(w204) -> ("Core.Close Panel on Exit?"=w203:bool)
        n71 = Select(t="UI: Front Panel State >> Close", s=w203, f="") -> (s? t:f=w200:string)
        n72 = call <vilib>:"Add State(s) to Queue__jki_lib_state_machine.vi"("State(s) in (\"\")"=w200, "State(s) at Back (\"\")"="Data: Cleanup\nExit") -> ("States Out"=w198:string)  [unwired: 13 in]
        n73 = call <vilib>:"Add State(s) to Queue__jki_lib_state_machine.vi"("State(s) in Front (\"\")"=w198, "State(s) in (\"\")"=w207) -> ("States Out"=w206:string)  [unwired: 13 in]
      }
      frame "---------- New Category ----------" {
        # "Template Separator\n(You can make a copy of, or modify, this frame)"
        n74 = call <vilib>:"Add State(s) to Queue__jki_lib_state_machine.vi"("State(s) in (\"\")"=w211) -> ("States Out"=w210:string)  [unwired: 14 in]
      }
      frame "SID4open" {
        # "Your code here.\n(You can make a copy of, or modify, this frame)"
        n75 = disable-structure shown="Enabled" {
          disable-tunnel: w216 -> [w234 _]
          disable-tunnel: [w221 _] -> w213
          disable-tunnel: [w219 _] -> w212
          frame Enabled {
            n76 = call "SDKSID4_Open SID4.vi"("Error code in"=w234, "User profile location"="Profile path") -> ("Error code out"=w222:errorcluster, "SDKSID4 sessionID"=w220:T12)  [unwired: 4 in]
            n77 = call "SDKSID4_Get User Profile.vi"("SDKSID4 session In"=w220, "error in"=w222) -> ("SDK Version"=→"SDKVersion":string, "UserProfileName"=→"UserProfileName":string, "UserProfile_File"=→"UserProfile_File":string, "UserProfileDescription"=→"UserProfileDescription":string, "UserProfile_LastReference"=→"UserProfile_LastReference":string, "SDKSID4 session Out"=w219:T12, "UserProfileDirectory"=→"UserProfileDirectory":string, "SNPhasics"=→"SNPhasics":string, "Analysis info"=→"Analysis info":T5, "Camera info"=→"Camera info":T6, "ImageCameraSize"=→"ImageCameraSize":T7, "error out"=w221:errorcluster)  [unwired: 14 in]
          }
          frame Disabled {
          }
        }
        n78 = Bundle By Name(cluster=w215, "SDKSID4 sessionID"=w212) -> (w214:T13)
        n79 = call <vilib>:"Add State(s) to Queue__jki_lib_state_machine.vi"("State(s) in (\"\")"=w218) -> ("States Out"=w217:string)  [unwired: 14 in]
      }
      frame "SID4analyze" {
        # "Your code here.\n(You can make a copy of, or modify, this frame)"
        n80 = Unbundle By Name(w245) -> ("Interferogram path"=w241:path, "SDKSID4 sessionID"=w247:T12)
        n81 = case shown="True" "file?" {
          tunnel: w247 -> [w250 w288]
          tunnel: w246 -> [w252 w292]
          tunnel: [w254 w291] -> w238
          tunnel: [w256 w290] -> w243
          tunnel: [w255 w286] -> _
          tunnel: w241 -> [w251 w287]
          tunnel: [w253 w285] -> w240
          frame False {
            n82 = disable-structure shown="Enabled" {
              disable-tunnel: [w266 w279] -> w256
              disable-tunnel: [w265 w280] -> w255
              disable-tunnel: [w264 w278] -> w254
              disable-tunnel: [w263 w277] -> w253
              disable-tunnel: w252 -> [w262 _]
              disable-tunnel: w251 -> [w260 _]
              disable-tunnel: w250 -> [w259 w283]
              frame Disabled {
                n83 = disable-structure shown="Enabled" {
                  disable-tunnel: w262 -> [w269 w272]
                  disable-tunnel: [w268 w273] -> w261
                  disable-tunnel: [w267 w274] -> w257
                  disable-tunnel: w260 -> [_ w276]
                  disable-tunnel: w259 -> [_ w275]
                  disable-tunnel: [_ w271] -> w258
                  frame Enabled {
                    n84 = call "IMAQ ImageToArray"("error in (no error)"=w269, "Image"=T3 refnum ("image::1")) -> ("error out"=w268:errorcluster, "Image Pixels (I16)"=w267:i16[][])  [unwired: 2 in, 3 out]
                  }
                  frame Disabled {
                    n85 = call "SDKSID4_Load Interferogram.vi"("SDKSID4 session In"=w275, "Interferogram File"=w276, "error in (no error)"=w272) -> ("SDKSID4 session Out"=w271:T12, "Interferogram[I16]"=w274:i16[][], "error out"=w273:errorcluster)  [unwired: 9 in, 1 out]
                  }
                }
                n86 = call "SDKSID4_Array Analysis.vi"("SDKSID4 session In"=w258, "Interferogram in (ArrayI16)"=w257, "error in (no error)"=w261) -> ("SDKSID4 session Out"=w265:T12, "Intensity out"=w266:sgl[][], "Phase out"=w264:sgl[][], "error out"=w263:errorcluster)  [unwired: 8 in, 1 out]
              }
              frame Enabled {
                n87 = call-poly "IMAQ Write File 2"("File Path"="Tmp path", "Image"=T3 refnum ("image::1")) -> ("error out"=w282:errorcluster)  [unwired: 8 in, 1 out]
                n88 = call "SDKSID4_File Analysis.vi"("SDKSID4 session In"=w283, "Interferogram File"="Tmp path", "error in (no error)"=w282) -> ("SDKSID4 session Out"=w280:T12, "Intensity out"=w279:sgl[][], "Phase out"=w278:sgl[][], "error out"=w277:errorcluster)  [unwired: 8 in, 1 out]
              }
            }
          }
          frame True {
            n89 = call "SID4analyzefile.vi"("error in (no error)"=w292, "Interferogram path"=w287, "Refnum in"=w288) -> ("error out"=w285:errorcluster, "Intensity out"=w290:sgl[][], "Image Out"=→"phasics-int1":T3, "Refnum out"=w286:T12, "Phase out"=w291:sgl[][])  [unwired: 4 in]
          }
        }
        "INTENSITY" <- w243
        "PHASE" <- w238
        n90 = Transpose 2D Array(2D array=w238) -> (transposed array=w235:sgl[][])
        n91 = call "IMAQ ArrayToImage"("Image Pixels (Float)"=w235, "Image"="phaseplot" ("Image Name")) -> ("Image Out"=→"phaseplot":T3)  [unwired: 8 in, 1 out]
        n92 = Bundle By Name(cluster=w245, "Interferogram path"=w241, "INTENSITY"=w243, "PHASE"=w238) -> (w244:T13)
        n93 = call <vilib>:"Add State(s) to Queue__jki_lib_state_machine.vi"("State(s) in Front (\"\")"="lineout" ("State(s) in Front (\"\")"), "State(s) in (\"\")"=w249) -> ("States Out"=w248:string)  [unwired: 13 in]
      }
      frame "SID4changereference" {
        # "Your code here.\n(You can make a copy of, or modify, this frame)"
        n94 = Unbundle By Name(w294) -> ("SDKSID4 sessionID"=w293:T12)
        n95 = call "SDKSID4_Change Reference.vi"("error in (no error)"=w296, "Reference path"="Reference Interferogram path", "Reference source"=enum16{"Workshop", "File", "Camera"}."File", "SDKSID4 session In"=w293) -> ("error out"=w295:errorcluster)  [unwired: 1 in, 2 out]
        n96 = call <vilib>:"Add State(s) to Queue__jki_lib_state_machine.vi"("State(s) in (\"\")"=w300) -> ("States Out"=w299:string)  [unwired: 14 in]
      }
      frame "SID4close" {
        # "Your code here.\n(You can make a copy of, or modify, this frame)"
        n97 = disable-structure shown="Enabled" {
          disable-tunnel: w303 -> [w309 _]
          disable-tunnel: w302 -> [w307 _]
          disable-tunnel: [w306 _] -> w301
          frame Enabled {
            n98 = Unbundle By Name(w309) -> ("SDKSID4 sessionID"=w308:T12)
            n99 = call "SDKSID4_Close SID4.vi"("error in (no error)"=w307, "SDKSID4 session In"=w308) -> ("error out"=w306:errorcluster)  [unwired: 4 in, 1 out]
          }
          frame Disabled {
          }
        }
        n100 = call <vilib>:"Add State(s) to Queue__jki_lib_state_machine.vi"("State(s) in (\"\")"=w305) -> ("States Out"=w304:string)  [unwired: 14 in]
      }
      frame "SID4changemask" {
        # "Your code here.\n(You can make a copy of, or modify, this frame)"
        n101 = Unbundle By Name(w315) -> ("SDKSID4 sessionID"=w314:T12)
        n102 = case shown="\"From control\"" "MASK" {
          tunnel: w312 -> [w322 w326 w331]
          tunnel: [w321 w324 w333] -> w311
          tunnel: w314 -> [w320 w325 w332]
          tunnel: [w318 w323 w334] -> w310
          frame "From file", Default {
            n103 = call "SDKSID4_Change Mask.vi"("error in (no error)"=w322, "Mask file"="Mask path", "SDKSID4 session In"=w320) -> ("error out"=w321:errorcluster, "ROI Descriptor Out"=w318:T1)  [unwired: 2 in, 1 out]
            n104 = property on="phasics-int1" class="ImageControl"("ROI"=w318) -> ()  [unwired: 2 in, 2 out]
          }
          frame "From descriptor" {
            n105 = call "SDKSID4_Change Mask.vi"("error in (no error)"=w326, "ROI Descriptor"="ROI Descriptor IN", "SDKSID4 session In"=w325) -> ("error out"=w324:errorcluster, "ROI Descriptor Out"=w323:T1)  [unwired: 2 in, 1 out]
          }
          frame "From control" {
            n106 = local read "file?"() -> (w328:bool)
            n107 = case shown="False" w328 {
              tunnel: w331 -> [w336 w340]
              tunnel: [w337 w339] -> w330
              tunnel: [w335 w338] -> w329
              frame False {
                n108 = property on="image::1" class="ImageControl"(error in=w336) -> (error out=w337:errorcluster, "ROI"=w335:T16)  [unwired: 1 in, 1 out]
              }
              frame True {
                n109 = property on="phasics-int1" class="ImageControl"(error in=w340) -> (error out=w339:errorcluster, "ROI"=w338:T16)  [unwired: 1 in, 1 out]
              }
            }
            n110 = call "SDKSID4_Change Mask.vi"("error in (no error)"=w330, "ROI Descriptor"=w329, "SDKSID4 session In"=w332) -> ("error out"=w333:errorcluster, "ROI Descriptor Out"=w334:T1)  [unwired: 2 in, 1 out]
          }
        }
        "ROI Descriptor out" <- w310
        n111 = call "roi divisible by 4.vi"("ROI Descriptor Out"=w310) -> ()  [unwired: 9 in, 2 out]
        n112 = call <vilib>:"Add State(s) to Queue__jki_lib_state_machine.vi"("State(s) in (\"\")"=w317) -> ("States Out"=w316:string)  [unwired: 14 in]
      }
      frame "SID4savemeasurement" {
        # "Your code here.\n(You can make a copy of, or modify, this frame)"
        n113 = Unbundle By Name(w349) -> ("PHASE"=w341:sgl[][], "SDKSID4 sessionID"=w348:T12, "Interferogram path"=w344:path, "INTENSITY"=w347:sgl[][])
        n114 = call "SID4 GEECS save measurement.vi"("PHASE"=w341, "error in (no error)"=w345, "INTENSITY"=w347, "Interferogram path"=w344, "Refnum in"=w348) -> ("error out"=w346:errorcluster, "Saved Phase file"=→"Saved Phase file":path, "Intensity file"=→"Intensity file":path)  [unwired: 4 in]
        n115 = call <vilib>:"Add State(s) to Queue__jki_lib_state_machine.vi"("State(s) in (\"\")"=w351) -> ("States Out"=w350:string)  [unwired: 14 in]
      }
      frame "SID4saveraw" {
        # "Your code here.\n(You can make a copy of, or modify, this frame)"
        n116 = call "File Dialog"() -> ("selected path"=w352:path, "cancelled"=w355:bool)  [unwired: 12 in, 2 out]
        n117 = case shown="False" w355 {
          tunnel: w354 -> [w361 w363]
          tunnel: [w360 w363] -> w353
          tunnel: w352 -> [w359 _]
          frame False {
            n118 = call-poly "IMAQ Write File 2"("error in (no error)"=w361, "File Path"=w359, "Image"=T3 refnum ("image::1")) -> ("error out"=w360:errorcluster)  [unwired: 7 in, 1 out]
          }
          frame True {
          }
        }
        n119 = call <vilib>:"Add State(s) to Queue__jki_lib_state_machine.vi"("State(s) in (\"\")"=w358) -> ("States Out"=w357:string)  [unwired: 14 in]
      }
      frame "LoopInit" {
        # "Your code here.\n(You can make a copy of, or modify, this frame)"
        n120 = List Folder(path="Folder to analyze", pattern="pattern") -> (path out=w367:path, filenames=w368:string[])  [unwired: 2 in, 2 out]
        "filenames" <- w368
        n121 = for {
          tunnel: w368 -> [w377] mode=indexing
          tunnel: w367 -> [w376]
          tunnel: [w375] -> w364 mode=indexing
          n122 = Build Path(base path=w376, name or relative path=w377) -> (appended path=w375:path)
        }
        n123 = Bundle By Name(cluster=w366, "File paths"=w364) -> (w365:T13)
        n124 = call <vilib>:"Add State(s) to Queue__jki_lib_state_machine.vi"("State(s) in (\"\")"=w374, "State(s) at Back (\"\")"="LoopLogic" ("State(s) at Back (\"\")")) -> ("States Out"=w373:string)  [unwired: 13 in]
      }
      frame "LoopLogic" {
        # "Your code here.\n(You can make a copy of, or modify, this frame)"
        n125 = Unbundle By Name(w380) -> ("File paths"=w381:path[])
        n126 = Array Size(array=w381) -> (size(s)=w383:i32)
        n127 = Equal To 0?(x=w383) -> (x = 0?=w382:bool)
        n128 = case shown="False" w382 {
          tunnel: w381 -> [w394 _]
          tunnel: w380 -> [w391 w395]
          tunnel: [w390 w395] -> w379
          tunnel: ["SID4analyze\nSID4savemeasurement\nLoopLogic" ("State(s) in Front (\"\")") _] -> w378
          frame False {
            n129 = Delete From Array(array=w394, length=1) -> (deleted portion=w392:path[], array with subset deleted=w387:path[])  [unwired: 1 in]
            n130 = Index Array(array=w392) -> (element=w388:path)  [unwired: 1 in]
            n131 = Bundle By Name(cluster=w391, "File paths"=w387, "Interferogram path"=w388) -> (w390:T13)
          }
          frame True {
          }
        }
        n132 = call <vilib>:"Add State(s) to Queue__jki_lib_state_machine.vi"("State(s) in (\"\")"=w386, "State(s) at Back (\"\")"=w378) -> ("States Out"=w385:string)  [unwired: 13 in]
      }
      frame "ChangeAdvParameters" {
        # "Your code here.\n(You can make a copy of, or modify, this frame)"
        n133 = Unbundle By Name(w399) -> ("SDKSID4 sessionID"=w398:T12)
        n134 = call "SDKSID4_ADV_Set Integration Param.vi"("SDKSID4 session In"=w398, "Adv_Activation"="Adv_Activation in", "Adv_Niter"="Adv_Niter 2", "Adv_MSE_Threshold"="Adv_MSE_Threshold 2", "error in (no error)"=w397) -> ("error out"=w410:errorcluster)  [unwired: 9 in, 1 out]
        n135 = call "SDKSID4_ADV_Set unwrap Param.vi"("SDKSID4 session In"=w398, "UnwrappingAlgoritm"="UnwrappingAlgoritm IN", "UnwrappingOptions"="UnwrappingOptions IN", "error in (no error)"=w397) -> ("error out"=w405:errorcluster)  [unwired: 10 in, 1 out]
        n136 = call "SDKSID4_ADV_Get Integration Param.vi"("SDKSID4 session In"=w398, "error in (no error)"=w410) -> ("Adv_Activation"=→"Adv_Activation out":bool, "Adv_Niter"=→"Adv_Niter":u16, "Adv_MSE_Threshold"=→"Adv_MSE_Threshold":sgl)  [unwired: 9 in, 2 out]
        n137 = call "SDKSID4_ADV_Get unwrap Param.vi"("SDKSID4 session In"=w398, "error in (no error)"=w405) -> ("SDKSID4 session Out"=w409:T12, "UnwrappingAlgoritm"=→"UnwrappingAlgoritm":u16, "UnwrappingOptions"=→"UnwrappingOptions":u8[], "error out"=w408:errorcluster)  [unwired: 10 in]
        n138 = call "SDKSID4_Save Current User Profile.vi"("error in (no error)"=w408, "SDKSID4 session In"=w409) -> ("error out"=w396:errorcluster)  [unwired: 4 in, 1 out]
        n139 = call <vilib>:"Add State(s) to Queue__jki_lib_state_machine.vi"("State(s) in (\"\")"=w415) -> ("States Out"=w414:string)  [unwired: 14 in]
      }
      frame "lineout" {
        # "Your code here.\n(You can make a copy of, or modify, this frame)"
        n140 = property on="phaseplot" class="ImageControl"() -> ("ROI"=w420:T16)  [unwired: 2 in, 2 out]
        n141 = Unbundle By Name(w420) -> ("Global Rectangle"=w416:i32[])
        n142 = call "IMAQ LineProfile"("error in (no error)"=w422, "Line Coordinates"=w416, "Image"="phaseplot" ("Image Name")) -> ("error out"=w421:errorcluster, "Line Graph"=→"Line Profile":cluster{"x0":sgl, "dx":sgl, "Pixels Line":sgl[]}, "Line Information"=→"Line Information":T17)  [unwired: 2 in, 1 out]
        n143 = call <vilib>:"Add State(s) to Queue__jki_lib_state_machine.vi"("State(s) in (\"\")"=w425) -> ("States Out"=w424:string)  [unwired: 14 in]
      }
      frame "ggg" {
        # "Your code here.\n(You can make a copy of, or modify, this frame)"
        n144 = call <vilib>:"Add State(s) to Queue__jki_lib_state_machine.vi"("State(s) in (\"\")"=w429) -> ("States Out"=w428:string)  [unwired: 14 in]
      }
    }
  }
  n145 = disable-structure shown="Disabled" {
    frame Disabled {
    }
    frame Enabled {
    }
  }
  n146 = Create User Event(user event datatype=T10 {"EventEnum"=enum."new data", "Device name"="Device name"} ("New Event")) -> (user event=w3:refnum<user-event>, error out=w4:errorcluster)  [unwired: 1 in]
  "tcp data event" <- w3
  n147 = register-events(w3) -> ()  [unwired: 2 in, 2 out]
  n148 = control-ref of="This Application"() -> (w2:refnum<vi>)
  n149 = control-ref of="This VI"() -> (w7:refnum<vi>)
  n150 = Current VI's Menubar() -> (w6:refnum<k9>)
  n151 = call "GUI_Master_subvi_reentrant_queues.vi"("This Application"=w2, "error in (no error)"=w4, "tcp data event"=w3, "Caller menu reference"=w6, "Caller VI ref"=w7) -> ("error out"=→"error IO 2":errorcluster)  [unwired: 6 in]
  "image::1" <- T3 refnum ("image::1")
